vi "Name Score.vi"(11 "Name":string) -> (3 "Name Score":i32)   [LabVIEW 2013, in "Problem 22.lvlib"]
uses:
  Problem 22.lvlib
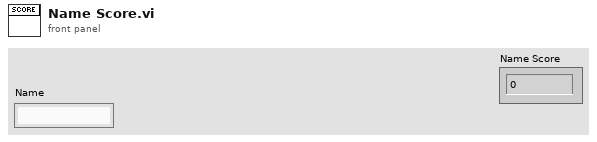
[diagram p1: front panel]
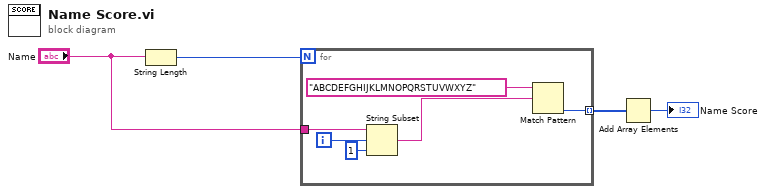
[diagram p0: block diagram]
diagram:
  n1 = String Length(string="Name") -> (length=w4:i32)
  n2 = for {
    N: w4 -> [_]
    tunnel: "Name" -> [w10]
    tunnel: [w5] -> w2 mode=indexing
    i -> [w9]
    n3 = String Subset(string=w10, offset (0)=w9, length (rest)=1 ("length (rest)")) -> (substring=w6:string)
    n4 = Match Pattern(string="ABCDEFGHIJKLMNOPQRSTUVWXYZ", regular expression=w6) -> (offset past match=w5:i32)  [unwired: 1 in, 3 out]
  }
  n5 = Add Array Elements(numeric array=w2) -> (sum=→"Name Score":i32)
